vi "Create ABORT.vi"(8 "error in (no error)":errorcluster, 10 "Abort Request":T3, 11 "WAMP Client in":refnum<class "WAMP Client.lvclass">) -> (0 "error out":errorcluster, 2 "Write queue item":T1, 3 "WAMP Client out":refnum<class "WAMP Client.lvclass">)   [LabVIEW 2020, in "wamplv.lvlib" / "WAMP Client.lvclass"]
uses:
  WAMP Client.lvclass
  WAMP Client.lvclass/WAMP Client.ctl
  Private/Requests/Abort/Abort JSON/Abort JSON.lvclass
  TypeDef/Termination Reason Enum.ctl
  API/TypeDefs/Termination Reason.ctl
  wamplv.lvlib
  Private/TypeDefs/Transport type.ctl
  TypeDef/Write queue item.ctl
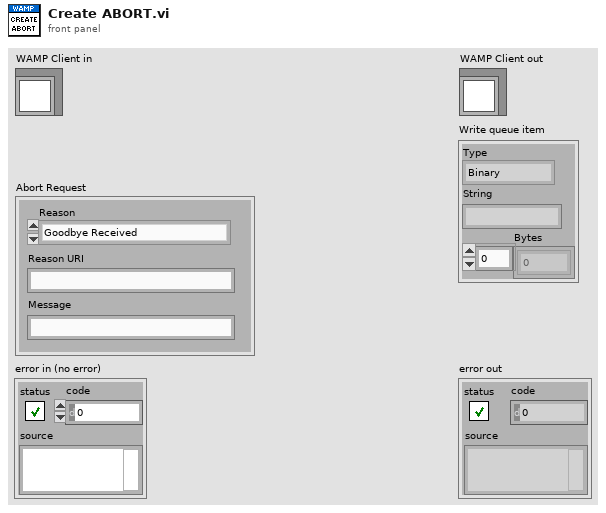
[diagram p1: front panel]
types:
  T1 = typedef "wamplv.lvlib/Write queue item.ctl" = cluster{"Type":T2, "String":string, "Bytes":u8[]}
  T2 = typedef "wamplv.lvlib/Transport type.ctl" = enum16{"Binary", "Text"}
  T3 = typedef "wamplv.lvlib/Termination Reason.ctl" = cluster{"Reason":T4, "Reason URI":string, "Message":string}
  T4 = typedef "wamplv.lvlib/WAMP Client.lvclass/Termination Reason Enum.ctl" = enum16{"Goodbye Received", "Abort Received", "Send Goodbye", "Send Abort", "Read Loop Failure", "Write Loop Failure", "Message Loop Failure", "wamplv aborted"}
  T5 = typedef "wamplv.lvlib/WAMP Client.lvclass/Serialisation.ctl" = enum16{"JSON", "MessagePack"}
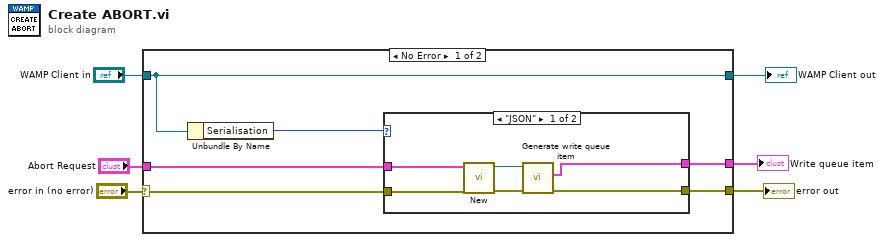
[diagram p0: block diagram]
diagram:
  n1 = case shown="No Error" "error in (no error)" {
    selector: "error in (no error)" -> [w10 w19]
    tunnel: "WAMP Client in" -> [w7 w20]
    tunnel: "Abort Request" -> [w11 _]
    tunnel: [w9 w19] -> w3
    tunnel: [w8 _] -> w2
    tunnel: [w7 w20] -> w1
    frame No Error {
      n2 = Unbundle By Name(w7) -> ("Serialisation"=w12:T5)
      n3 = case shown="\"JSON\"" w12 {
        tunnel: w11 -> [w18 _]
        tunnel: w10 -> [w14 _]
        tunnel: [w15 _] -> w9
        tunnel: [w13 _] -> w8
        frame "JSON" {
          n4 = call "New.vi"("error in (no error)"=w14, "Termination Reason"=w18) -> ("error out"=w17:errorcluster, "Abort JSON out"=w16:refnum<class "Abort JSON.lvclass">)  [unwired: 8 in]
          n5 = call-dynamic "Generate write queue item.vi"("error in (no error)"=w17, "Abort JSON in"=w16) -> ("error out"=w15:errorcluster, "Write queue item"=w13:T1)  [unwired: 7 in, 1 out]
        }
        frame "MessagePack" {
        }
      }
    }
    frame Error {
    }
  }
  "error out" <- w3
  "WAMP Client out" <- w1
  "Write queue item" <- w2
